vi "demo - first while loop.vi"() -> ()   [LabVIEW 2024]
doc: "#vi_description \nPlot a sine wave onto a waveform chart\nThetic Engineering Ltd."
panel:
  in  "Stop":bool
  out "Waveform Chart":dbl(graph)
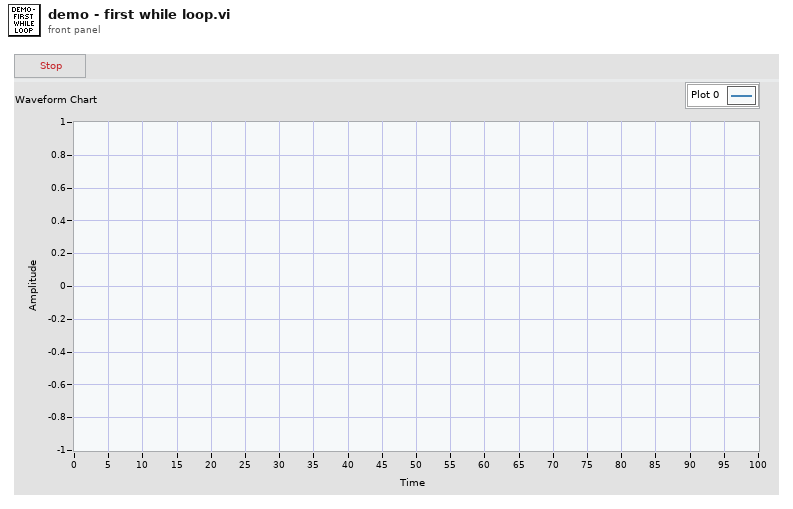
[diagram p1: front panel]
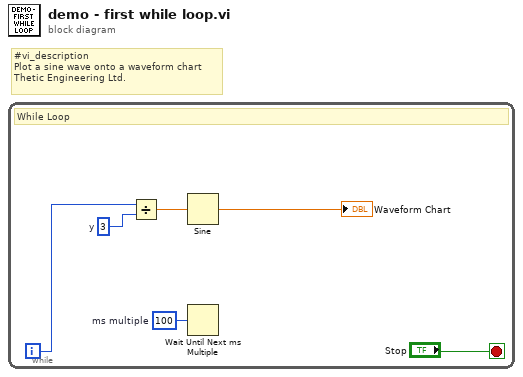
[diagram p0: block diagram]
diagram:
  # "#vi_description \nPlot a sine wave onto a waveform chart\nThetic Engineering Ltd."
  n1 = while {
    i -> [w4]
    stop <- "Stop" stop-if-true
    w1 = u32 100  # ms multiple
    w2 = 3  # y
    # "While Loop"
    n2 = Divide(x=w4, y=w2) -> (x/y=w3:dbl)
    n3 = Sine(x=w3) -> (sin(x)=→"Waveform Chart":dbl)
    n4 = Wait Until Next ms Multiple(millisecond multiple=w1) -> ()  [unwired: 1 out]
  }
